vi "HeaderAction.vi"(0 "InstrClass":refnum<class "DAQ6363.lvclass"> caption="DNL_LabVIEW Object in", 11 "error in (no error)":errorcluster caption="entrée d'erreur (pas d'erreur)") -> (4 "InstrClassOut":refnum<class "DAQ6363.lvclass"> caption="DNL_LabVIEW Object out", 6 "DataNames":string[](array[string]), 8 "Instr Name":string, 10 "HeaderString":string, 13 "ArrDisplayNames":string[](array[string]), 14 "DisplayNames":string[](array[string]), 15 "error out":errorcluster caption="sortie d'erreur")   [LabVIEW 2019, in "DAQ6363.lvclass"]
uses:
  DAQ6363.lvclass
  C:/Programmes Labview/LabscanV1A/DevicesClass/BaseDevice/BaseDevice.lvclass
  DAQ6363.lvclass/DAQ6363.ctl
  <userlib>/GenProg/ReadValByRefTask.vi
  <userlib>/GenProg/ReadValByRefBool.vi
  <userlib>/GenProg/ReadValByRefU32.vi
  <userlib>/GenProg/ReadValByRefDbl.vi
  <userlib>/GenProg/ReadValByRefI32.vi
  BaseDevice/BaseDevice.lvclass
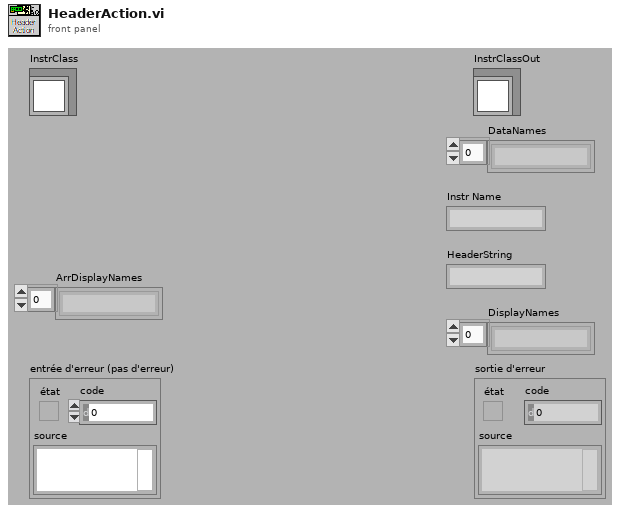
[diagram p1: front panel]
types:
  T1 = typedef "DAQ6363.lvclass/DAQ6363_Func.ctl" = enum16{"CountPulse (Cnt)", "Rabi (Tau)", "MWtoLaserDelay (us)", "APDGate (us)", "PulsedODMR (Pulses)", "PulsedODMR_AWG (Pulses)", "DiffPulsedODMR_AWG (Pulses)", "DiffPulsedODMR (Pulses)"}
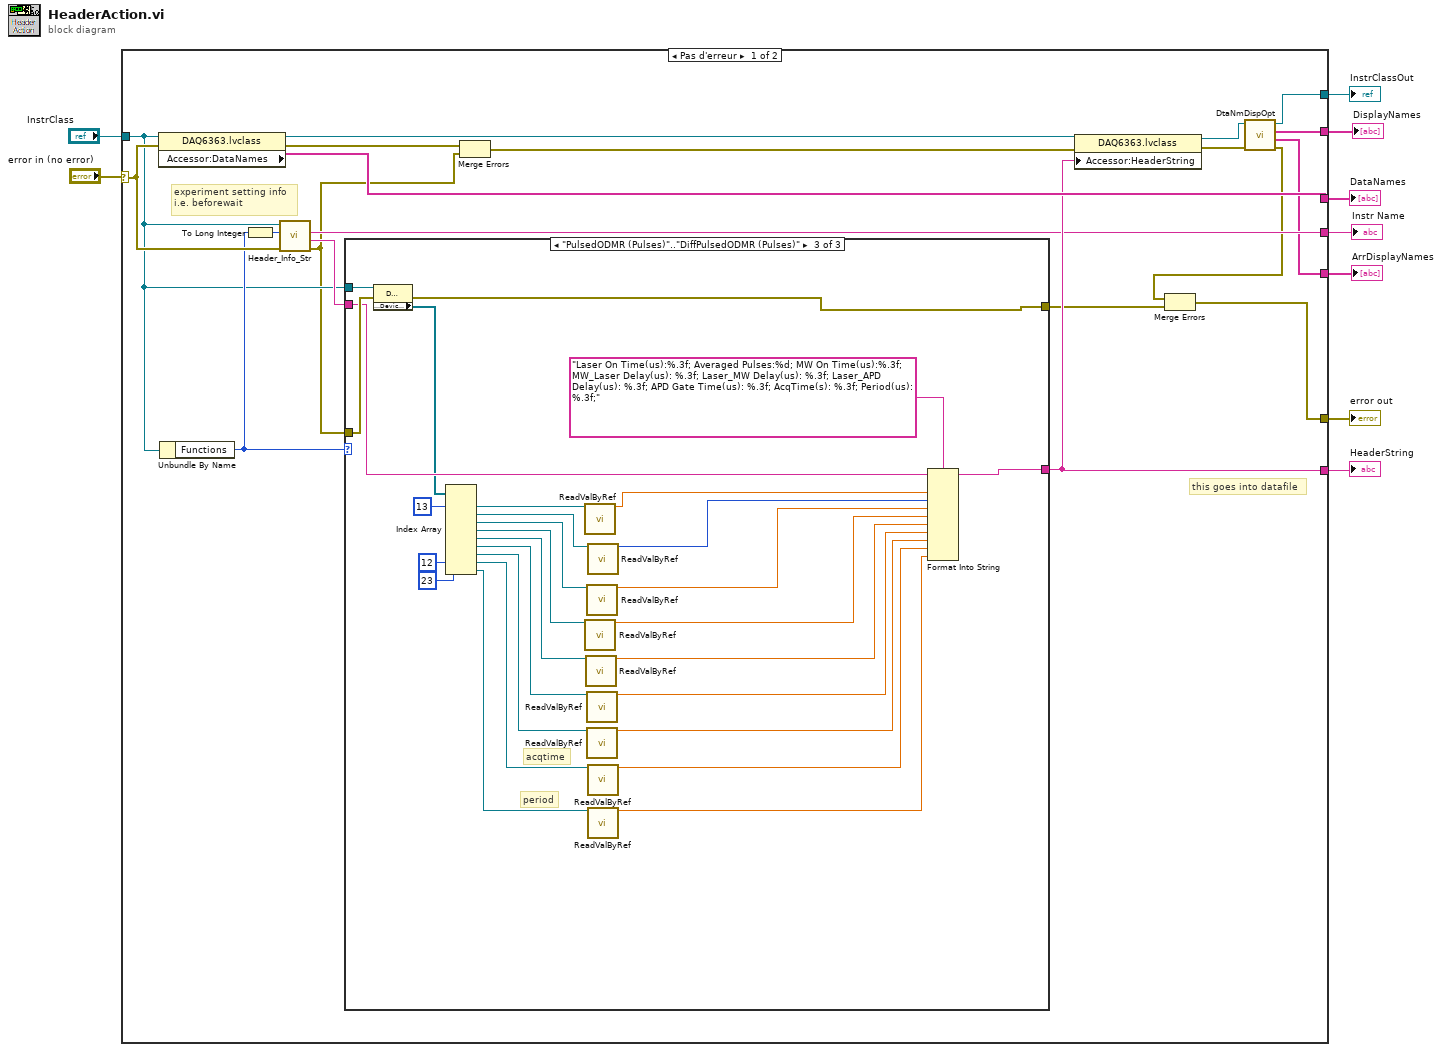
[diagram p0: block diagram]
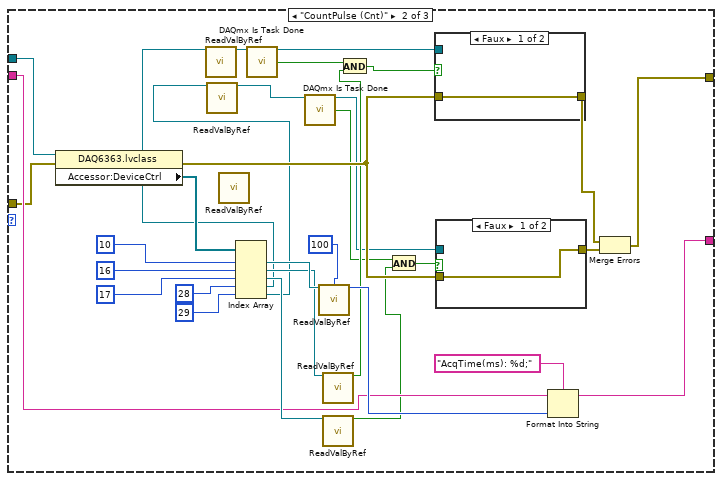
[diagram p3: hidden frame]
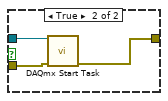
[diagram p4: hidden frame]
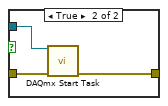
[diagram p5: hidden frame]
diagram:
  n1 = case shown="Pas d'erreur" "error in (no error)" {
    selector: "error in (no error)" -> [w19 w100]
    tunnel: [w26 _] -> w8
    tunnel: [w29 _] -> w7
    tunnel: "InstrClass" -> [w14 w101]
    tunnel: [w10 w100] -> w5
    tunnel: [w24 w101] -> w3
    tunnel: [w21 _] -> w4
    tunnel: [w22 _] -> w2
    tunnel: [w15 _] -> w1
    frame No Error {
      # "this goes into datafile"
      # "experiment setting info\ni.e. beforewait"
      n2 = property class="DAQ6363.lvclass"(reference=w14, error in=w19) -> (reference out=w28:refnum<class "DAQ6363.lvclass">, error out=w27:errorcluster, "Accessor:DataNames"=w29:string[])
      n3 = Unbundle By Name(w14) -> ("Functions"=w17:T1)
      n4 = To Long Integer(number=w17) -> (32bit integer=w16:i32)
      n5 = call-dynamic "Header_Info_Str.vi"("error in (no error)"=w19, "Functions"=w16, "DefaultDev in"=w14) -> ("error out"=w13:errorcluster, "HdrInfoStr"=w20:string, "InstrumentName"=w21:string)  [unwired: 5 in, 1 out]
      n6 = case shown="\"PulsedODMR (Pulses)\"..\"DiffPulsedODMR (Pulses)\"" w17 {
        tunnel: [w31 w51 w95] -> w26
        tunnel: w20 -> [w31 w52 w96]
        tunnel: w14 -> [_ w63 w99]
        tunnel: w13 -> [w30 w50 w98]
        tunnel: [w30 w46 w81] -> w12
        frame Default {
        }
        frame "CountPulse (Cnt)" {
          n7 = property class="DAQ6363.lvclass"(reference=w63, error in=w50) -> (error out=w49:errorcluster, "Accessor:DeviceCtrl"=w59:refnum<vi>[])  [unwired: 1 out]
          n8 = call-poly <userlib>:"ReadValByRef.vi"() -> ()  [unwired: 14 in, 2 out]
          n9 = Index Array(array=w59, index #1=10 ("indice"), index #2=16 ("indice"), index #3=17 ("indice"), index #4=28 ("indice"), index #5=29 ("indice")) -> (element #1=w57:refnum<vi>, element #2=w56:refnum<vi>, element #3=w55:refnum<vi>, element #4=w35:refnum<vi>, element #5=w34:refnum<vi>)
          n10 = call-poly <userlib>:"ReadValByRef.vi"("Control Ref"=w35) -> ("Valeur"=w37:refnum<k21>)  [unwired: 13 in, 1 out]
          n11 = call-poly <userlib>:"ReadValByRef.vi"("Control Ref"=w34) -> ("Valeur"=w36:refnum<k21>)  [unwired: 13 in, 1 out]
          n12 = call <vilib>:"DAQmx Is Task Done.vi"("task/channels in"=w37) -> ("task out"=w45:refnum<k21>, "task done?"=w44:bool)  [unwired: 12 in, 1 out]
          n13 = call <vilib>:"DAQmx Is Task Done.vi"("task/channels in"=w36) -> ("task out"=w41:refnum<k21>, "task done?"=w38:bool)  [unwired: 12 in, 1 out]
          n14 = call-poly <userlib>:"ReadValByRef.vi"("Control Ref"=w57, "Type In"=u32 100 ("Count Period (ms)")) -> ("Valeur"=w53:u32)  [unwired: 12 in, 1 out]
          n15 = call-poly <userlib>:"ReadValByRef.vi"("Control Ref"=w56) -> ("Valeur"=w43:bool)  [unwired: 13 in, 1 out]
          n16 = call-poly <userlib>:"ReadValByRef.vi"("Control Ref"=w55) -> ("Valeur"=w40:bool)  [unwired: 13 in, 1 out]
          n17 = And(x=w44, y=w43) -> (x .and. y?=w42:bool)
          n18 = And(x=w38, y=w40) -> (x .and. y?=w39:bool)
          n19 = case shown="Faux" w42 {
            tunnel: w45 -> [_ w71]
            tunnel: w49 -> [w68 w70]
            tunnel: [w68 w69] -> w47
            frame False {
            }
            frame True {
              n20 = call <vilib>:"DAQmx Start Task.vi"("task/channels in"=w71, "error in"=w70) -> ("error out"=w69:errorcluster)  [unwired: 12 in, 1 out]
            }
          }
          n21 = case shown="Faux" w39 {
            tunnel: w41 -> [_ w67]
            tunnel: w49 -> [w64 w66]
            tunnel: [w64 w65] -> w48
            frame False {
            }
            frame True {
              n22 = call <vilib>:"DAQmx Start Task.vi"("task/channels in"=w67, "error in"=w66) -> ("error out"=w65:errorcluster)  [unwired: 12 in, 1 out]
            }
          }
          n23 = Format Into String(format string="AcqTime(ms): %d;" ("chaîne de format"), initial string=w52, w53) -> (resulting string=w51:string)  [unwired: 1 in, 1 out]
          n24 = Merge Errors(w47, w48) -> (w46:errorcluster)
        }
        frame "PulsedODMR (Pulses)".."DiffPulsedODMR (Pulses)" {
          # "acqtime"
          # "period"
          n25 = property class="DAQ6363.lvclass"(reference=w99, error in=w98) -> (error out=w81:errorcluster, "Accessor:DeviceCtrl"=w94:refnum<vi>[])  [unwired: 1 out]
          n26 = Index Array(array=w94, index #1=13 ("indice"), index #8=12 ("indice"), index #9=23 ("indice")) -> (element #1=w93:refnum<vi>, element #2=w82:refnum<vi>, element #3=w75:refnum<vi>, element #4=w74:refnum<vi>, element #5=w91:refnum<vi>, element #6=w89:refnum<vi>, element #7=w88:refnum<vi>, element #8=w87:refnum<vi>, element #9=w77:refnum<vi>)  [unwired: 6 in]
          n27 = call-poly <userlib>:"ReadValByRef.vi"("Control Ref"=w93) -> ("Valeur"=w92:dbl)  [unwired: 13 in, 1 out]
          n28 = call-poly <userlib>:"ReadValByRef.vi"("Control Ref"=w74) -> ("Valeur"=w72:dbl)  [unwired: 13 in, 1 out]
          n29 = call-poly <userlib>:"ReadValByRef.vi"("Control Ref"=w91) -> ("Valeur"=w90:dbl)  [unwired: 13 in, 1 out]
          n30 = call-poly <userlib>:"ReadValByRef.vi"("Control Ref"=w75) -> ("Valeur"=w73:dbl)  [unwired: 13 in, 1 out]
          n31 = call-poly <userlib>:"ReadValByRef.vi"("Control Ref"=w89) -> ("Valeur"=w86:dbl)  [unwired: 13 in, 1 out]
          n32 = call-poly <userlib>:"ReadValByRef.vi"("Control Ref"=w88) -> ("Valeur"=w85:dbl)  [unwired: 13 in, 1 out]
          n33 = call-poly <userlib>:"ReadValByRef.vi"("Control Ref"=w82) -> ("Valeur"=w76:i32)  [unwired: 13 in, 1 out]
          n34 = call-poly <userlib>:"ReadValByRef.vi"("Control Ref"=w87) -> ("Valeur"=w84:dbl)  [unwired: 13 in, 1 out]
          n35 = call-poly <userlib>:"ReadValByRef.vi"("Control Ref"=w77) -> ("Valeur"=w78:dbl)  [unwired: 13 in, 1 out]
          n36 = Format Into String(format string="Laser On Time(us):%.3f; Averaged Pulses:%d; MW On Time(us):%.3f;  MW_Laser Delay(us): %.3f; Laser_MW Delay(us): %.3f; Laser_APD Delay(us): %.3f; APD Gate Time(us): %.3f; AcqTime(s): %.3f; Period(us): %.3f;" ("chaîne de format"), initial string=w96, w92, w76, w73, w72, w90, w86, w85, w84, w78) -> (resulting string=w95:string)  [unwired: 1 in, 1 out]
        }
      }
      n37 = Merge Errors(w27, w13) -> (w18:errorcluster)
      n38 = property class="DAQ6363.lvclass"(reference=w28, error in=w18, "Accessor:HeaderString"=w26) -> (reference out=w23:refnum<class "DAQ6363.lvclass">, error out=w25:errorcluster)
      n39 = call "DtaNmDispOpt.vi"("error in (no error)"=w25, "BaseDevice en entrée"=w23) -> ("error out"=w11:errorcluster, "ArrDisplayNames"=w15:string[], "DisplayNames"=w22:string[], "BaseDevice en sortie"=w24:refnum<class "DAQ6363.lvclass">)  [unwired: 6 in]
      n40 = Merge Errors(w11, w12) -> (w10:errorcluster)
    }
    frame Error {
    }
  }
  "error out" <- w5
  "InstrClassOut" <- w3
  "DataNames" <- w7
  "HeaderString" <- w8
  "Instr Name" <- w4
  "DisplayNames" <- w2
  "ArrDisplayNames" <- w1
